vi "LabVIEW Hiss [2021-04-01].vi"() -> ()   [LabVIEW 2020]
uses:
  States [2021-04-01].ctl
panel:
  in  "?":enum32{"Hisspanel", "Inställningar"}(tab)
  in  "Våningar":T1
  out "Lampor":T2
  in  "?":bool
  out "Målvärde":dbl
  out "Våningstolerans, Ohm":dbl
  out "Våningshöjd, Ohm":dbl
  in  "Meta nödstopp":bool
  in  "GPIB-addresser":T3={"Funktionsgenerator"="1", "Multimeter"="3", "Nätaggregat"="2"}
  in  "Antal våningar":i32=5
  in  "Tolerans relativt \nvåningshöjd.\n1 -> 100%\n5 -> 20%":i32=5
  in  "Potentiometerinställningar":T4
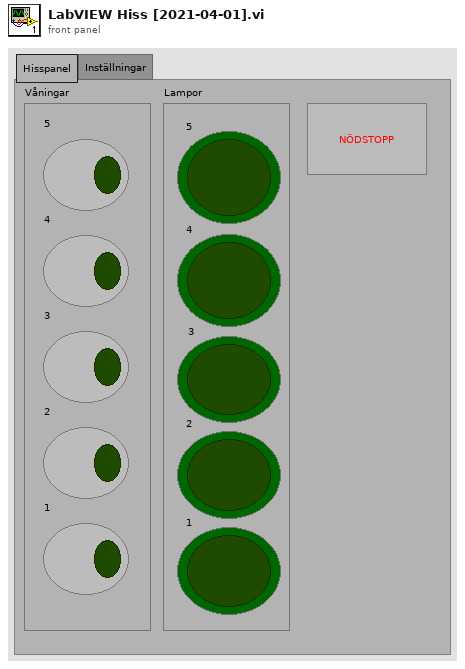
[diagram p1: front panel]
types:
  T1 = cluster{"1":bool, "2":bool, "3":bool, "4":bool, "5":bool}
  T2 = cluster{"1":bool, "\n2":bool, "3":bool, "4":bool, "5":bool}
  T3 = cluster{"Funktionsgenerator":string, "Multimeter":string, "Nätaggregat":string}
  T4 = cluster{"Högsta våning":dbl, "Lägsta våning":dbl}
  T5 = cluster{"Våningshöjd":dbl, "Våningstolerans":dbl, "Högsta våning":dbl, "Lägsta våning":dbl}
  T6 = typedef "States [2021-04-01].ctl" = enum16{"Initialtillstånd", "Kör ner", "Kör upp", "Vänta på input", "Spela ljudfil", "Nödstopp"}
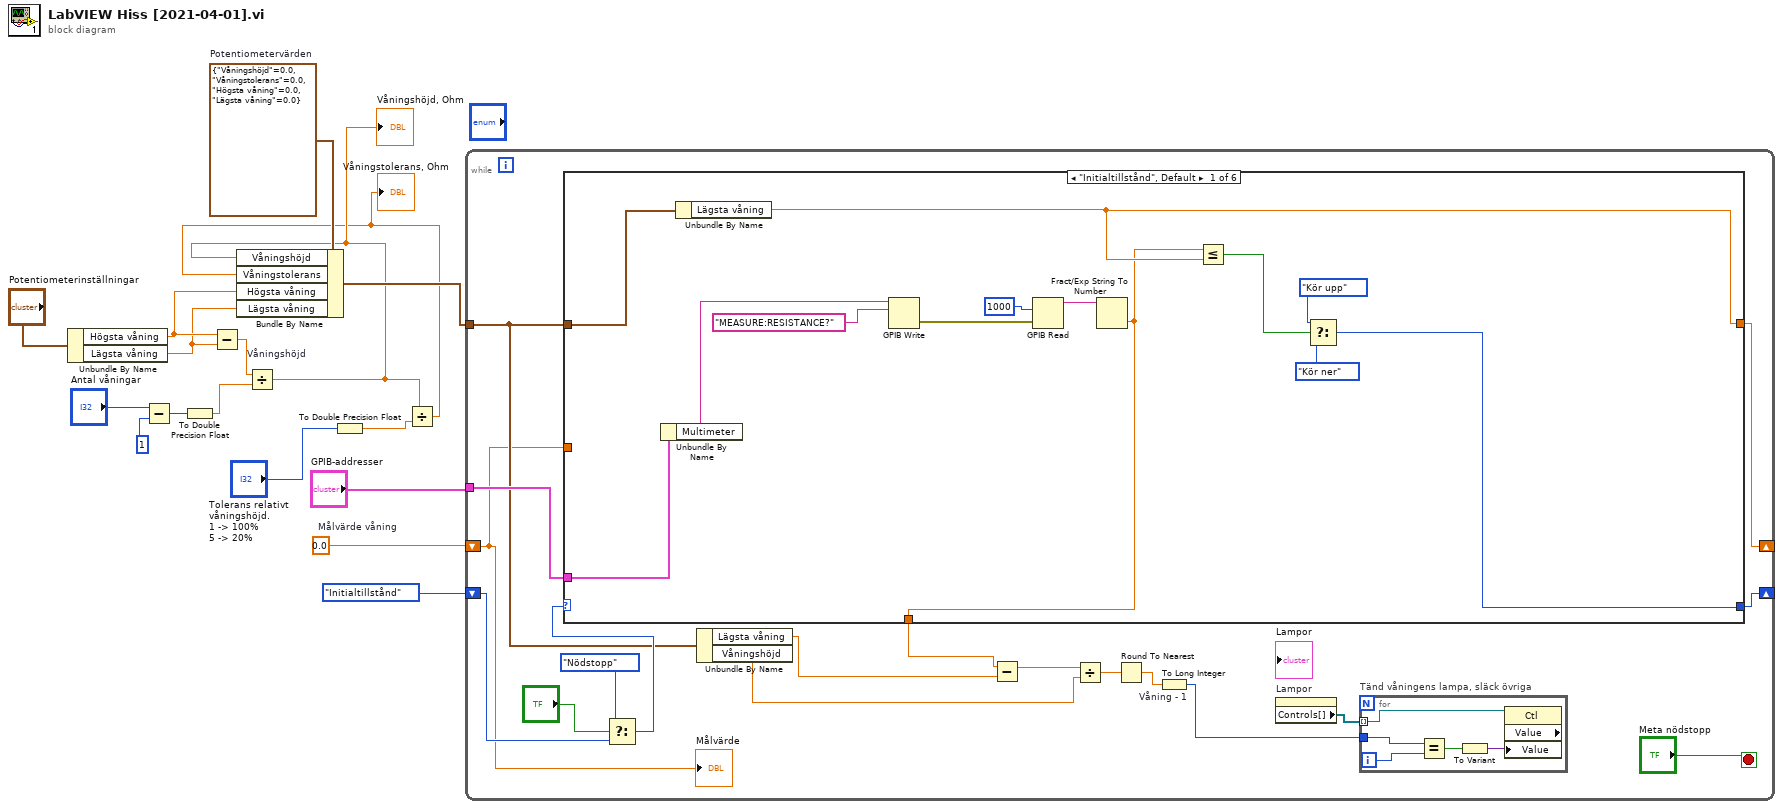
[diagram p0: block diagram]
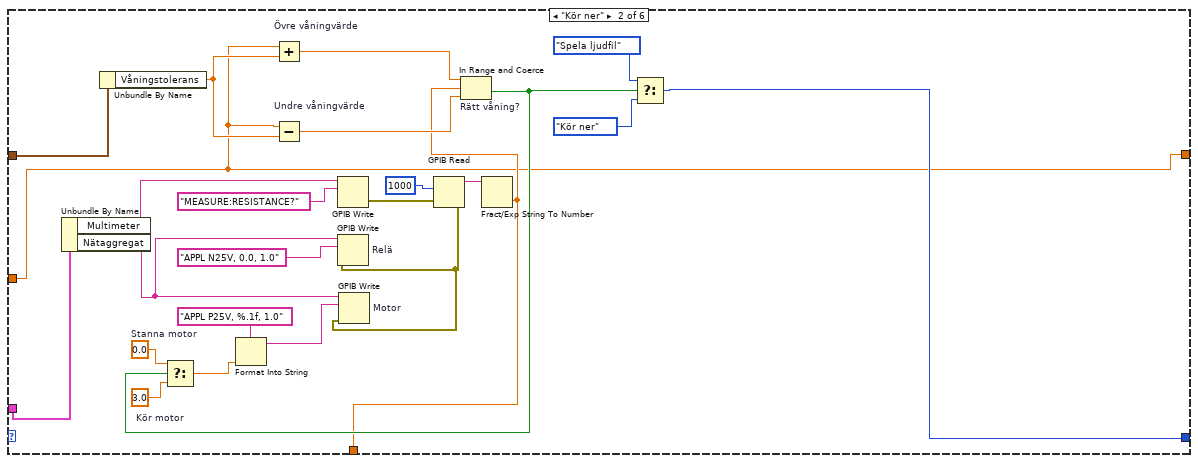
[diagram p2: hidden frame]
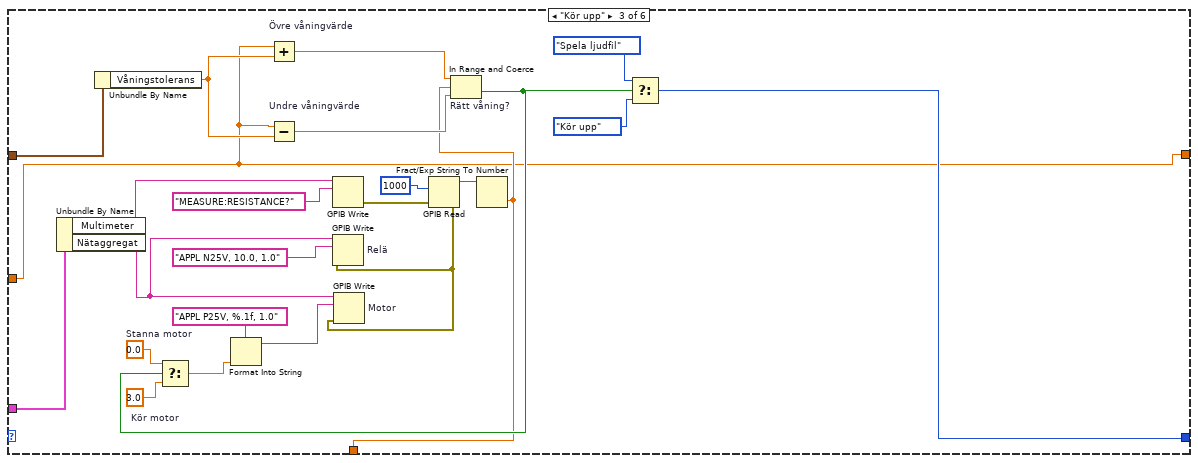
[diagram p3: hidden frame]
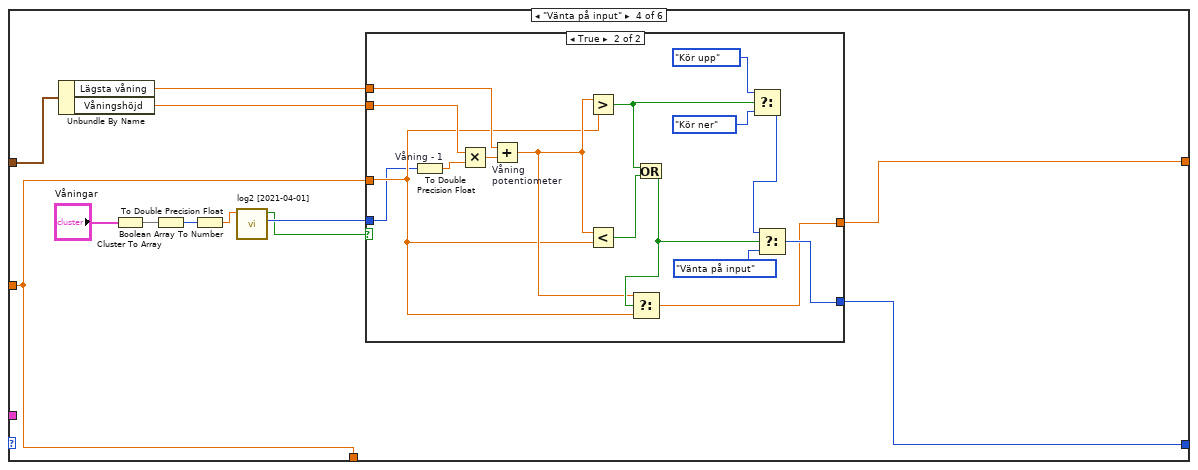
[diagram p4: hidden frame]
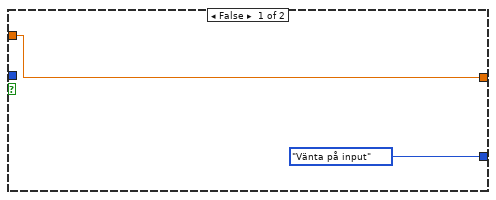
[diagram p5: hidden frame]
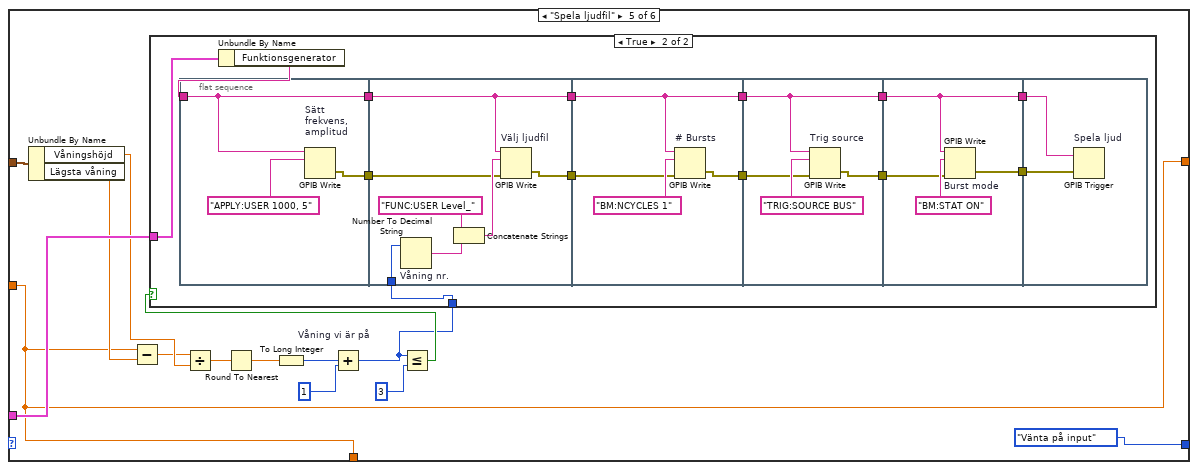
[diagram p6: hidden frame]
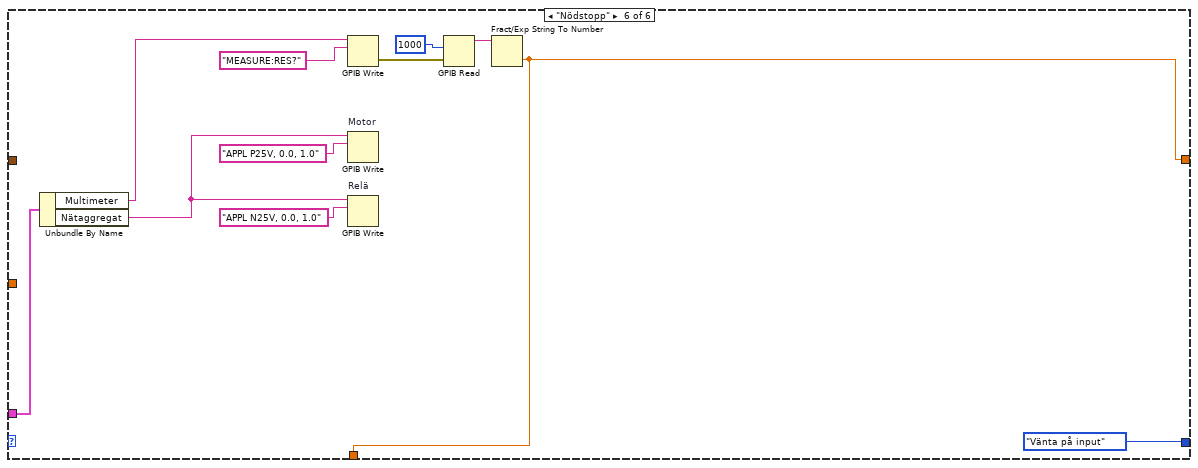
[diagram p8: hidden frame]
diagram:
  w16 = 0.0  # Målvärde våning
  w10 = T5 {"Våningshöjd"=0.0, "Våningstolerans"=0.0, "Högsta våning"=0.0, "Lägsta våning"=0.0}  # Potentiometervärden
  n1 = Unbundle By Name("Potentiometerinställningar") -> ("Högsta våning"=w3:dbl, "Lägsta våning"=w2:dbl)
  n2 = Subtract(x="Antal våningar", y=1) -> (x-y=w13:i32)
  n3 = To Double Precision Float(number=w13) -> (double precision float=w12:dbl)
  n4 = Subtract(x=w3, y=w2) -> (x-y=w14:dbl)
  n5 = Divide "Våningshöjd"(x=w14, y=w12) -> (x/y=w7:dbl)
  "Våningshöjd, Ohm" <- w7
  n6 = To Double Precision Float(number="Tolerans relativt \nvåningshöjd.\n1 -> 100%\n5 -> 20%") -> (double precision float=w11:dbl)
  n7 = Divide(x=w7, y=w11) -> (x/y=w6:dbl)
  "Våningstolerans, Ohm" <- w6
  n8 = Bundle By Name(cluster=w10, "Våningshöjd"=w7, "Våningstolerans"=w6, "Högsta våning"=w3, "Lägsta våning"=w2) -> (w9:T5)
  n9 = while {
    shift-right: [w30] -> _
    shift-left: States_[2021-04-01]."Initialtillstånd" -> [w34]
    tunnel: "GPIB-addresser" -> [w31]
    shift-right: [w29] -> _
    shift-left: w16 -> [w18]
    tunnel: w9 -> [w23]
    stop <- "Meta nödstopp" stop-if-true
    n10 = Select(t=States_[2021-04-01]."Nödstopp", s="?", f=w34) -> (s? t:f=w32:T6)
    n11 = case shown="\"Initialtillstånd\", Default" w32 {
      tunnel: w31 -> [w53 w58 w83 _ w145 w193]
      tunnel: [w44 w57 w82 w108 States_[2021-04-01]."Vänta på input" States_[2021-04-01]."Vänta på input"] -> w30
      tunnel: [w43 w55 w78 w107 w132 w183] -> w29
      tunnel: w23 -> [w42 w59 w84 w111 w144 _]
      tunnel: w18 -> [_ w55 w78 w103 w132 _]
      tunnel: [w41 w56 w81 w103 w132 w183] -> w24
      frame "Initialtillstånd", Default {
        n12 = Unbundle By Name(w53) -> ("Multimeter"=w52:string)
        n13 = Unbundle By Name(w42) -> ("Lägsta våning"=w43:dbl)
        n14 = GPIB Write(0:w52, 1:"MEASURE:RESISTANCE?") -> (6:w50:errorcluster)  [unwired: 3 in, 1 out]
        n15 = GPIB Read(1:1000, 3:w50) -> (5:w48:string)  [unwired: 3 in, 2 out]
        n16 = Fract/Exp String To Number(string=w48) -> (number=w41:dbl)  [unwired: 3 in, 1 out]
        n17 = Less Or Equal?(x=w41, y=w43) -> (x <= y?=w47:bool)
        n18 = Select(t=States_[2021-04-01]."Kör upp", s=w47, f=States_[2021-04-01]."Kör ner") -> (s? t:f=w44:T6)
      }
      frame "Kör ner" {
        w67 = 3.0  # Kör motor
        w68 = 0.0  # Stanna motor
        n19 = Unbundle By Name(w58) -> ("Multimeter"=w60:string, "Nätaggregat"=w65:string)
        n20 = Unbundle By Name(w59) -> ("Våningstolerans"=w73:dbl)
        n21 = Add "Övre våningvärde"(x=w55, y=w73) -> (x+y=w72:dbl)
        n22 = Subtract "Undre våningvärde"(x=w55, y=w73) -> (x-y=w71:dbl)
        n23 = GPIB Write(0:w60, 1:"MEASURE:RESISTANCE?") -> (6:w76:errorcluster)  [unwired: 3 in, 1 out]
        n24 = GPIB Read(1:1000, 3:w76) -> (5:w74:string, 7:w54:errorcluster)  [unwired: 3 in, 1 out]
        n25 = GPIB Write "Relä"(0:w65, 1:"APPL N25V, 0.0, 1.0", 3:w54) -> ()  [unwired: 2 in, 2 out]
        n26 = Fract/Exp String To Number(string=w74) -> (number=w56:dbl)  [unwired: 3 in, 1 out]
        n27 = In Range and Coerce "Rätt våning?"(upper limit=w72, x=w56, lower limit=w71) -> (In Range?=w61:bool)  [unwired: 1 out]
        n28 = Select(t=w68, s=w61, f=w67) -> (s? t:f=w66:dbl)
        n29 = Format Into String(format string="APPL P25V, %.1f, 1.0", w66) -> (resulting string=w69:string)  [unwired: 2 in, 1 out]
        n30 = GPIB Write "Motor"(0:w65, 1:w69, 3:w54) -> ()  [unwired: 2 in, 2 out]
        n31 = Select(t=States_[2021-04-01]."Spela ljudfil", s=w61, f=States_[2021-04-01]."Kör ner") -> (s? t:f=w57:T6)
      }
      frame "Kör upp" {
        w91 = 3.0  # Kör motor
        w92 = 0.0  # Stanna motor
        n32 = Unbundle By Name(w83) -> ("Multimeter"=w80:string, "Nätaggregat"=w89:string)
        n33 = Unbundle By Name(w84) -> ("Våningstolerans"=w97:dbl)
        n34 = Add "Övre våningvärde"(x=w78, y=w97) -> (x+y=w96:dbl)
        n35 = Subtract "Undre våningvärde"(x=w78, y=w97) -> (x-y=w95:dbl)
        n36 = GPIB Write(0:w80, 1:"MEASURE:RESISTANCE?") -> (6:w100:errorcluster)  [unwired: 3 in, 1 out]
        n37 = GPIB Read(1:1000, 3:w100) -> (5:w98:string, 7:w79:errorcluster)  [unwired: 3 in, 1 out]
        n38 = GPIB Write "Relä"(0:w89, 1:"APPL N25V, 10.0, 1.0", 3:w79) -> ()  [unwired: 2 in, 2 out]
        n39 = Fract/Exp String To Number(string=w98) -> (number=w81:dbl)  [unwired: 3 in, 1 out]
        n40 = In Range and Coerce "Rätt våning?"(upper limit=w96, x=w81, lower limit=w95) -> (In Range?=w85:bool)  [unwired: 1 out]
        n41 = Select(t=w92, s=w85, f=w91) -> (s? t:f=w90:dbl)
        n42 = Format Into String(format string="APPL P25V, %.1f, 1.0", w90) -> (resulting string=w93:string)  [unwired: 2 in, 1 out]
        n43 = GPIB Write "Motor"(0:w89, 1:w93, 3:w79) -> ()  [unwired: 2 in, 2 out]
        n44 = Select(t=States_[2021-04-01]."Spela ljudfil", s=w85, f=States_[2021-04-01]."Kör upp") -> (s? t:f=w82:T6)
      }
      frame "Vänta på input" {
        n45 = Unbundle By Name(w111) -> ("Lägsta våning"=w109:dbl, "Våningshöjd"=w110:dbl)
        n46 = Cluster To Array(cluster="Våningar") -> (array=w102:bool[])
        n47 = Boolean Array To Number(Boolean array=w102) -> (number=w112:u32)
        n48 = To Double Precision Float(number=w112) -> (double precision float=w106:dbl)
        n49 = call "log2 [2021-04-01].vi"("Input"=w106) -> ("Numeric"=w105:i32, "Boolean"=w104:bool)  [unwired: 9 in]
        n50 = case shown="True" w104 {
          tunnel: w110 -> [_ w131]
          tunnel: w109 -> [_ w129]
          tunnel: [States_[2021-04-01]."Vänta på input" w122] -> w108
          tunnel: w103 -> [w115 w118]
          tunnel: [w115 w119] -> w107
          tunnel: w105 -> [_ w116]
          frame False {
          }
          frame True {
            n51 = To Double Precision Float "Våning - 1"(number=w116) -> (double precision float=w117:dbl)
            n52 = Multiply(x=w131, y=w117) -> (x*y=w130:dbl)
            n53 = Add "Våning\npotentiometer"(x=w129, y=w130) -> (x+y=w120:dbl)
            n54 = Greater?(x=w120, y=w118) -> (0:w127:bool)
            n55 = Less?(x=w120, y=w118) -> (x < y?=w128:bool)
            n56 = Or(x=w127, y=w128) -> (x .or. y?=w121:bool)
            n57 = Select(t=w120, s=w121, f=w118) -> (s? t:f=w119:dbl)
            n58 = Select(t=States_[2021-04-01]."Kör upp", s=w127, f=States_[2021-04-01]."Kör ner") -> (s? t:f=w123:T6)
            n59 = Select(t=w123, s=w121, f=States_[2021-04-01]."Vänta på input") -> (s? t:f=w122:T6)
          }
        }
      }
      frame "Spela ljudfil" {
        n60 = Unbundle By Name(w144) -> ("Våningshöjd"=w142:dbl, "Lägsta våning"=w143:dbl)
        n61 = Subtract(x=w132, y=w143) -> (x-y=w141:dbl)
        n62 = Divide(x=w141, y=w142) -> (x/y=w140:dbl)
        n63 = Round To Nearest(number=w140) -> (nearest integer value=w139:dbl)
        n64 = To Long Integer(number=w139) -> (32bit integer=w138:i32)
        n65 = Add "Våning vi är på"(x=w138, y=1) -> (x+y=w133:i32)
        n66 = Less Or Equal?(x=w133, y=3) -> (x <= y?=w135:bool)
        n67 = case shown="True" w135 {
          tunnel: w145 -> [_ w158]
          tunnel: w133 -> [_ w151]
          frame False {
          }
          frame True {
            n68 = flat-sequence {
              tunnel: w157 -> [w160]
              tunnel: [w160] -> w156
              tunnel: [w159] -> w150
              tunnel: w156 -> [w164]
              tunnel: w151 -> [w168]
              tunnel: [w164] -> w155
              tunnel: w150 -> [w163]
              tunnel: [w162] -> w149
              tunnel: w155 -> [w172]
              tunnel: [w172] -> w154
              tunnel: w149 -> [w170]
              tunnel: [w169] -> w148
              tunnel: w154 -> [w176]
              tunnel: [w176] -> w153
              tunnel: w148 -> [w174]
              tunnel: [w173] -> w147
              tunnel: w153 -> [w180]
              tunnel: [w180] -> w152
              tunnel: w147 -> [w178]
              tunnel: [w177] -> w146
              tunnel: w152 -> [w182]
              tunnel: w146 -> [w181]
              frame #0 {
                n69 = GPIB Write "Sätt\nfrekvens,\namplitud"(0:w160, 1:"APPLY:USER 1000, 5") -> (6:w159:errorcluster)  [unwired: 3 in, 1 out]
              }
              frame #1 {
                n70 = Number To Decimal String "Våning nr."(number=w168) -> (decimal integer string=w166:string)  [unwired: 1 in]
                n71 = Concatenate Strings("FUNC:USER Level_", w166) -> (w165:string)
                n72 = GPIB Write "Välj ljudfil"(0:w164, 1:w165, 3:w163) -> (6:w162:errorcluster)  [unwired: 2 in, 1 out]
              }
              frame #2 {
                n73 = GPIB Write "# Bursts"(0:w172, 1:"BM:NCYCLES 1", 3:w170) -> (6:w169:errorcluster)  [unwired: 2 in, 1 out]
              }
              frame #3 {
                n74 = GPIB Write "Trig source"(0:w176, 1:"TRIG:SOURCE BUS", 3:w174) -> (6:w173:errorcluster)  [unwired: 2 in, 1 out]
              }
              frame #4 {
                n75 = GPIB Write "Burst mode"(0:w180, 1:"BM:STAT ON", 3:w178) -> (6:w177:errorcluster)  [unwired: 2 in, 1 out]
              }
              frame #5 {
                n76 = GPIB Trigger "Spela ljud"(2:w181, 3:w182) -> ()  [unwired: 2 out]
              }
            }
            n77 = Unbundle By Name(w158) -> ("Funktionsgenerator"=w157:string)
          }
        }
      }
      frame "Nödstopp" {
        n78 = Unbundle By Name(w193) -> ("Multimeter"=w184:string, "Nätaggregat"=w190:string)
        n79 = GPIB Write(0:w184, 1:"MEASURE:RES?") -> (6:w188:errorcluster)  [unwired: 3 in, 1 out]
        n80 = GPIB Write "Motor"(0:w190, 1:"APPL P25V, 0.0, 1.0") -> ()  [unwired: 3 in, 2 out]
        n81 = GPIB Write "Relä"(0:w190, 1:"APPL N25V, 0.0, 1.0") -> ()  [unwired: 3 in, 2 out]
        n82 = GPIB Read(1:1000, 3:w188) -> (5:w186:string)  [unwired: 3 in, 2 out]
        n83 = Fract/Exp String To Number(string=w186) -> (number=w183:dbl)  [unwired: 3 in, 1 out]
      }
    }
    n84 = Unbundle By Name(w23) -> ("Lägsta våning"=w22:dbl, "Våningshöjd"=w21:dbl)
    n85 = Subtract(x=w24, y=w22) -> (x-y=w27:dbl)
    n86 = Divide(x=w27, y=w21) -> (x/y=w26:dbl)
    n87 = Round To Nearest(number=w26) -> (nearest integer value=w25:dbl)
    n88 = To Long Integer "Våning - 1"(number=w25) -> (32bit integer=w20:i32)
    n89 = property on="Lampor" class="Clust (strict)"() -> ("Controls[]"=w19:refnum<vi>[])  [unwired: 2 in, 2 out]
    n90 = for "Tänd våningens lampa, släck övriga" {
      tunnel: w20 -> [w39]
      tunnel: w19 -> [w40] mode=indexing
      i -> [w38]
      n91 = Equal?(x=w39, y=w38) -> (x = y?=w36:bool)
      n92 = To Variant(anything=w36) -> (Variant=w37:variant)
      n93 = property class="Ctl" props=["Value", "Value"](reference=w40, "Value"=w37) -> ()  [unwired: 1 in, 3 out]
    }
    "Målvärde" <- w18
  }
